vi "CREATE ITEM SQL QUERY.vi"(0 "What to Search":string, 5 "Search Column Name":string, 7 "Sorting Column Name":string, 9 "Column to Search In":u16, 11 "Column to Sort By":u16, 12 "Date Range":u16(ring) items=["Greater Than", "Less Than", "Between"], 13 "Dates Less Than":string="8/1/2023", 14 "Dates Greater Than":string="8/1/2023") -> (4 "SQL QUERY":string)   [LabVIEW 2019]
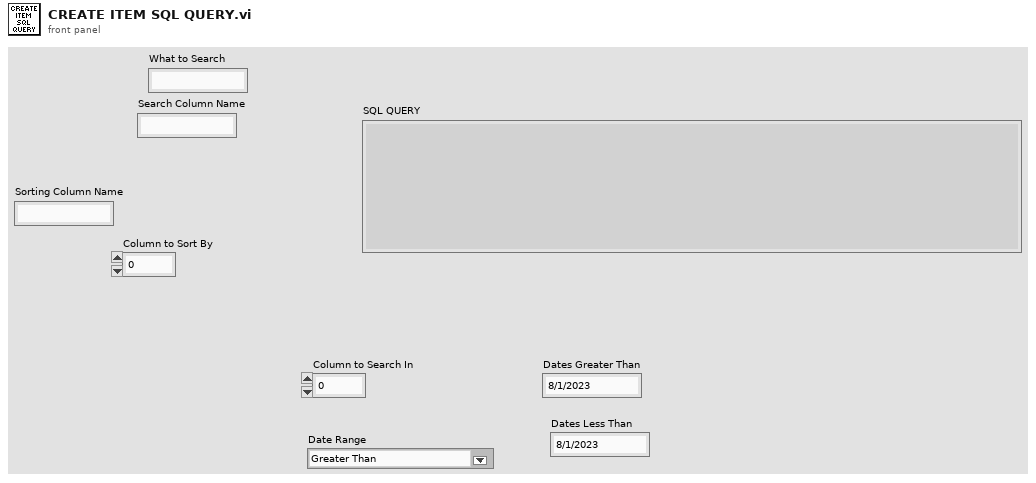
[diagram p1: front panel]
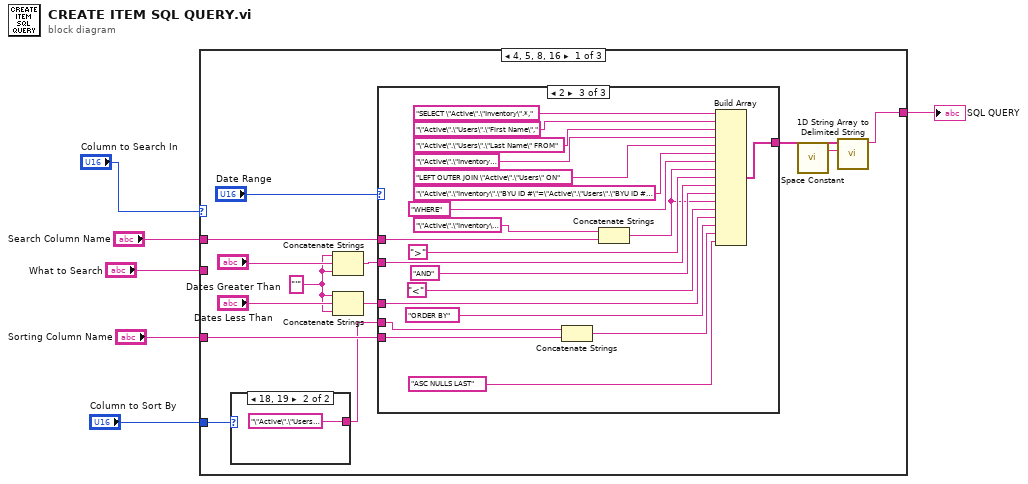
[diagram p0: block diagram]
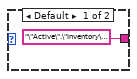
[diagram p2: hidden frame]
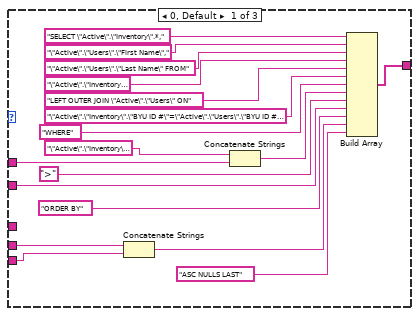
[diagram p3: hidden frame]
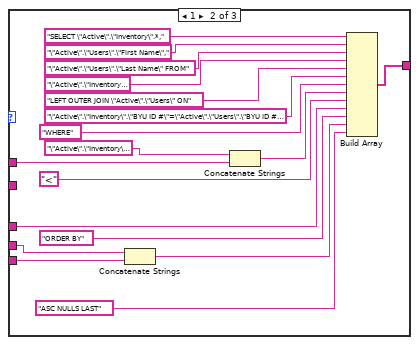
[diagram p4: hidden frame]
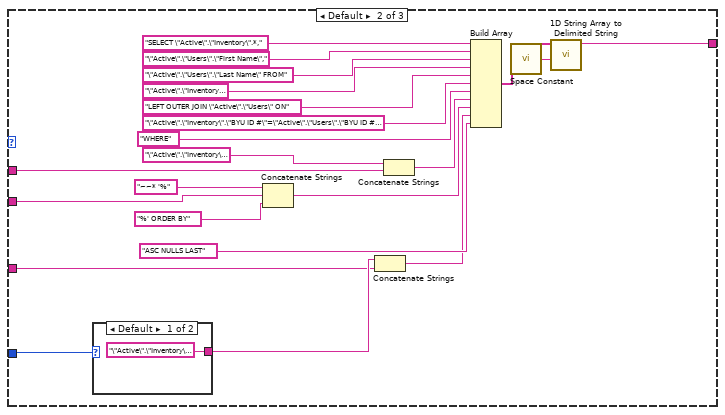
[diagram p5: hidden frame]
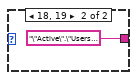
[diagram p6: hidden frame]
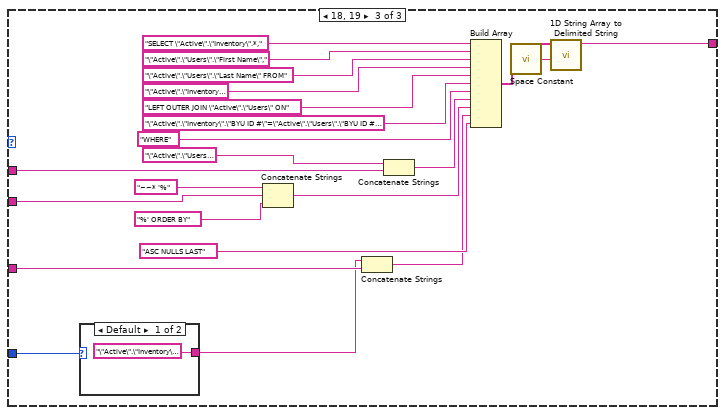
[diagram p7: hidden frame]
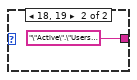
[diagram p8: hidden frame]
diagram:
  n1 = case shown="4, 5, 8, 16" "Column to Search In" {
    tunnel: "Search Column Name" -> [w19 w85 w109]
    tunnel: "Sorting Column Name" -> [w17 w81 w105]
    tunnel: [w15 w84 w108] -> w3
    tunnel: "What to Search" -> [_ w83 w107]
    tunnel: "Column to Sort By" -> [w8 w79 w106]
    frame 4, 5, 8, 16 {
      w9 = "'" ("string")
      n2 = case shown="18, 19" w8 {
        tunnel: ["\"Active\".\"Inventory\"." ("string") "\"Active\".\"Users\"." ("string")] -> w7
        frame Default {
        }
        frame 18, 19 {
        }
      }
      n3 = Concatenate Strings(w9, "Dates Greater Than", w9) -> (w13:string)
      n4 = Concatenate Strings(w9, "Dates Less Than", w9) -> (w12:string)
      n5 = case shown="2" "Date Range" {
        tunnel: w19 -> [w31 w49 w70]
        tunnel: w13 -> [w28 _ w68]
        tunnel: w17 -> [w23 w41 w59]
        tunnel: [w25 w43 w61] -> w16
        tunnel: w12 -> [_ w46 w64]
        tunnel: w7 -> [w24 w42 w60]
        frame 0, Default {
          n6 = Concatenate Strings(w24, w23) -> (w22:string)
          n7 = Concatenate Strings("\"Active\".\"Inventory\"." ("string"), w31) -> (w30:string)
          n8 = Build Array("SELECT \"Active\".\"Inventory\".*," ("string"), "\"Active\".\"Users\".\"First Name\"," ("string"), "\"Active\".\"Users\".\"Last Name\" FROM" ("string"), "\"Active\".\"Inventory\"" ("string"), "LEFT OUTER JOIN \"Active\".\"Users\" ON" ("string"), "\"Active\".\"Inventory\".\"BYU ID #\"=\"Active\".\"Users\".\"BYU ID #\"" ("string"), "WHERE" ("string"), w30, ">" ("string"), w28, "ORDER BY" ("string"), w22, "ASC NULLS LAST" ("string")) -> (w25:string[])
        }
        frame 1 {
          n9 = Concatenate Strings(w42, w41) -> (w40:string)
          n10 = Concatenate Strings("\"Active\".\"Inventory\"." ("string"), w49) -> (w48:string)
          n11 = Build Array("SELECT \"Active\".\"Inventory\".*," ("string"), "\"Active\".\"Users\".\"First Name\"," ("string"), "\"Active\".\"Users\".\"Last Name\" FROM" ("string"), "\"Active\".\"Inventory\"" ("string"), "LEFT OUTER JOIN \"Active\".\"Users\" ON" ("string"), "\"Active\".\"Inventory\".\"BYU ID #\"=\"Active\".\"Users\".\"BYU ID #\"" ("string"), "WHERE" ("string"), w48, "<" ("string"), w46, "ORDER BY" ("string"), w40, "ASC NULLS LAST" ("string")) -> (w43:string[])
        }
        frame 2 {
          n12 = Concatenate Strings(w60, w59) -> (w58:string)
          n13 = Concatenate Strings("\"Active\".\"Inventory\"." ("string"), w70) -> (w66:string)
          n14 = Build Array("SELECT \"Active\".\"Inventory\".*," ("string"), "\"Active\".\"Users\".\"First Name\"," ("string"), "\"Active\".\"Users\".\"Last Name\" FROM" ("string"), "\"Active\".\"Inventory\"" ("string"), "LEFT OUTER JOIN \"Active\".\"Users\" ON" ("string"), "\"Active\".\"Inventory\".\"BYU ID #\"=\"Active\".\"Users\".\"BYU ID #\"" ("string"), "WHERE" ("string"), w66, ">" ("string"), w68, "AND" ("string"), w66, "<" ("string"), w64, "ORDER BY" ("string"), w58, "ASC NULLS LAST" ("string")) -> (w61:string[])
        }
      }
      n15 = call <vilib>:"Space Constant.vi"() -> ("String"=w14:string)
      n16 = call <vilib>:"1D String Array to Delimited String.vi"("delimiter"=w14, "string array"=w16) -> ("delimited string"=w15:string)  [unwired: 9 in]
    }
    frame Default {
      n17 = case shown="Default" w79 {
        tunnel: ["\"Active\".\"Inventory\"." ("string") "\"Active\".\"Users\"." ("string")] -> w82
        frame Default {
        }
        frame 18, 19 {
        }
      }
      n18 = Concatenate Strings("~~* '%" ("string"), w83, "%' ORDER BY" ("string")) -> (w94:string)
      n19 = Concatenate Strings(w82, w81) -> (w80:string)
      n20 = Concatenate Strings("\"Active\".\"Inventory\"." ("string"), w85) -> (w86:string)
      n21 = Build Array("SELECT \"Active\".\"Inventory\".*," ("string"), "\"Active\".\"Users\".\"First Name\"," ("string"), "\"Active\".\"Users\".\"Last Name\" FROM" ("string"), "\"Active\".\"Inventory\"" ("string"), "LEFT OUTER JOIN \"Active\".\"Users\" ON" ("string"), "\"Active\".\"Inventory\".\"BYU ID #\"=\"Active\".\"Users\".\"BYU ID #\"" ("string"), "WHERE" ("string"), w86, w94, w80, "ASC NULLS LAST" ("string")) -> (w99:string[])
      n22 = call <vilib>:"Space Constant.vi"() -> ("String"=w100:string)
      n23 = call <vilib>:"1D String Array to Delimited String.vi"("delimiter"=w100, "string array"=w99) -> ("delimited string"=w84:string)  [unwired: 9 in]
    }
    frame 18, 19 {
      n24 = case shown="Default" w106 {
        tunnel: ["\"Active\".\"Inventory\"." ("string") "\"Active\".\"Users\"." ("string")] -> w104
        frame Default {
        }
        frame 18, 19 {
        }
      }
      n25 = Concatenate Strings("~~* '%" ("string"), w107, "%' ORDER BY" ("string")) -> (w118:string)
      n26 = Concatenate Strings(w104, w105) -> (w103:string)
      n27 = Concatenate Strings("\"Active\".\"Users\"." ("string"), w109) -> (w110:string)
      n28 = Build Array("SELECT \"Active\".\"Inventory\".*," ("string"), "\"Active\".\"Users\".\"First Name\"," ("string"), "\"Active\".\"Users\".\"Last Name\" FROM" ("string"), "\"Active\".\"Inventory\"" ("string"), "LEFT OUTER JOIN \"Active\".\"Users\" ON" ("string"), "\"Active\".\"Inventory\".\"BYU ID #\"=\"Active\".\"Users\".\"BYU ID #\"" ("string"), "WHERE" ("string"), w110, w118, w103, "ASC NULLS LAST" ("string")) -> (w123:string[])
      n29 = call <vilib>:"Space Constant.vi"() -> ("String"=w124:string)
      n30 = call <vilib>:"1D String Array to Delimited String.vi"("delimiter"=w124, "string array"=w123) -> ("delimited string"=w108:string)  [unwired: 9 in]
    }
  }
  "SQL QUERY" <- w3
